vi "DXYN.vi"(11 "Variables and Memory in":T1 {"GFX" format="%02x"}) -> (3 "Variables and Memory out":T1 {"GFX" format="%02x"})   [LabVIEW 2021]
uses:
  Controls/ClusterF.ctl
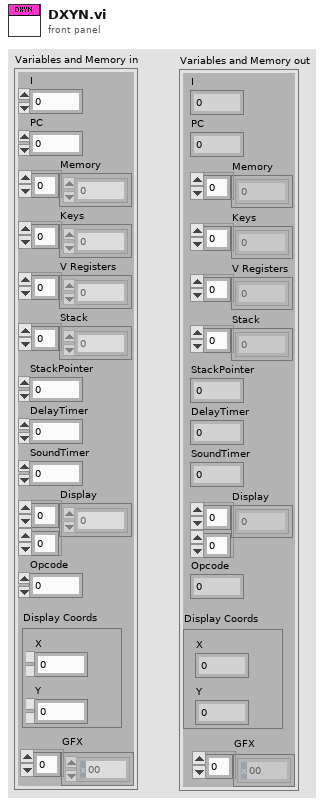
[diagram p1: front panel]
types:
  T1 = typedef "ClusterF.ctl" = cluster{"I":u16, "PC":u16, "Memory":u8[], "Keys":u8[], "V Registers":u8[], "Stack":u16[], "StackPointer":u16, "DelayTimer":u8, "SoundTimer":u8, "Display":u8[][], "Opcode":u16, "Display Coords":cluster{"X":u8, "Y":u8}, "GFX":u8[]}
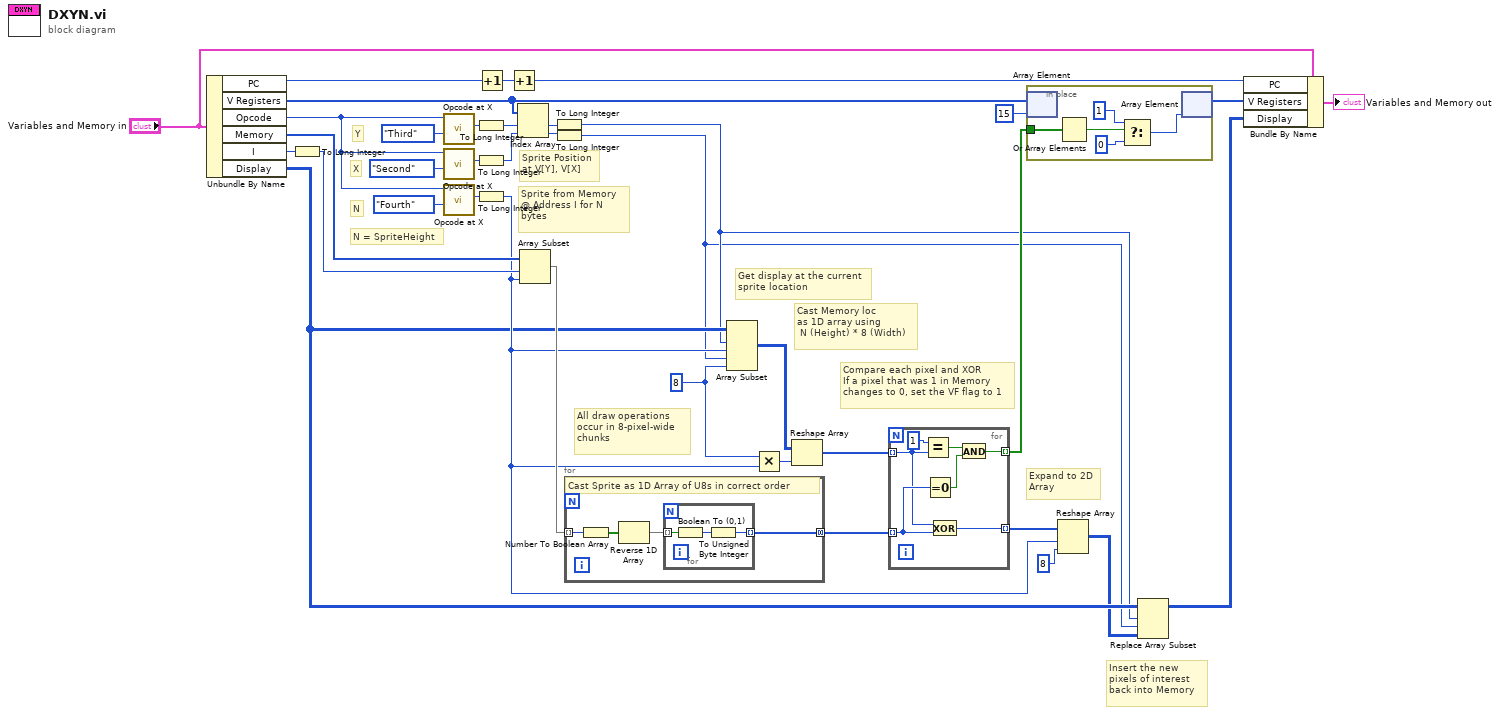
[diagram p0: block diagram]
diagram:
  w13 = 8 ("length")
  # "Insert the new\npixels of interest\nback into Memory"
  # "Expand to 2D\nArray"
  # "Compare each pixel and XOR\nIf a pixel that was 1 in Memory\nchanges to 0, set the VF flag to 1"
  # "Cast Memory loc \nas 1D array using\n N (Height) * 8 (Width)"
  # "Get display at the current\nsprite location"
  # "All draw operations\noccur in 8-pixel-wide\nchunks"
  # "Sprite Position\nat V[Y], V[X]"
  # "Sprite from Memory\n@ Address I for N\nbytes"
  # "N = SpriteHeight"
  # "N"
  # "X"
  # "Y"
  n1 = Unbundle By Name("Variables and Memory in") -> ("PC"=w24:u16, "V Registers"=w29:u8[], "Opcode"=w32:u16, "Memory"=w21:u8[], "I"=w20:u16, "Display"=w5:u8[][])
  n2 = To Long Integer(number=w20) -> (32bit integer=w19:i32)
  n3 = call "Opcode at X.vi"("X Position"=enum16{"First", "Second", "Third", "Fourth"}."Third", "Opcode"=w32) -> ("Opcode at X Position (U8)"=w28:u8)  [unwired: 9 in]
  n4 = call "Opcode at X.vi"("X Position"=enum16{"First", "Second", "Third", "Fourth"}."Second", "Opcode"=w32) -> ("Opcode at X Position (U8)"=w26:u8)  [unwired: 9 in]
  n5 = call "Opcode at X.vi"("X Position"=enum16{"First", "Second", "Third", "Fourth"}."Fourth", "Opcode"=w32) -> ("Opcode at X Position (U8)"=w18:u8)  [unwired: 9 in]
  n6 = To Long Integer(number=w28) -> (32bit integer=w27:i32)
  n7 = To Long Integer(number=w26) -> (32bit integer=w25:i32)
  n8 = To Long Integer(number=w18) -> (32bit integer=w7:i32)
  n9 = Increment(x=w24) -> (x+1=w22:u16)
  n10 = Increment(x=w22) -> (x+1=w23:u16)
  n11 = Index Array(array=w29, index #1=w27, index #2=w25) -> (element #1=w17:u8, element #2=w16:u8)
  n12 = Array Subset(array=w21, index=w19, length=w7) -> (w15:u8[])
  n13 = To Long Integer(number=w17) -> (32bit integer=w4:i32)
  n14 = To Long Integer(number=w16) -> (32bit integer=w3:i32)
  n15 = for {
    tunnel: w15 -> [w41] mode=indexing
    tunnel: [w38] -> w10 mode=concatenating
    # "Cast Sprite as 1D Array of U8s in correct order"
    n16 = Number To Boolean Array(number=w41) -> (Boolean array=w40:bool[])
    n17 = Reverse 1D Array(array=w40) -> (reversed array=w39:bool[])
    n18 = for {
      tunnel: w39 -> [w44] mode=indexing
      tunnel: [w42] -> w38 mode=indexing
      n19 = Boolean To (0,1)(Boolean=w44) -> (0, 1=w43:i16)
      n20 = To Unsigned Byte Integer(number=w43) -> (unsigned 8bit integer=w42:u8)
    }
  }
  n21 = Array Subset(array=w5, index (row)=w4, length (row)=w7, index (col)=w3, length (col)=w13) -> (w14:u8[][])
  n22 = Multiply(x=w13, y=w7) -> (x*y=w12:i32)
  n23 = Reshape Array(w14, w12) -> (w11:u8[])
  n24 = for {
    tunnel: w11 -> [w49] mode=indexing
    tunnel: w10 -> [w50] mode=indexing
    tunnel: [w46] -> w9 mode=indexing
    tunnel: [w45] -> w8 mode=indexing
    n25 = Equal?(x=u8 1, y=w49) -> (x = y?=w48:bool)
    n26 = Equal To 0?(x=w50) -> (x = 0?=w47:bool)
    n27 = Exclusive Or(1:w50, 2:w49) -> (0:w45:u8)
    n28 = And(x=w48, y=w47) -> (x .and. y?=w46:bool)
  }
  n29 = in-place {
    in-place-border: w9 -> [w52]
    n30 = in-place-array #1(w29, 15) -> ()  [unwired: 1 out]
    n31 = Or Array Elements(Boolean array=w52) -> (logical OR=w53:bool)
    n32 = Select(t=u8 1, s=w53, f=u8 0 ("element")) -> (s? t:f=w54:u8)
    n33 = in-place-array #1(w54) -> (w30:u8[])  [unwired: 1 out]
  }
  n34 = Reshape Array(w8, w7, 8 ("dimension size")) -> (w2:u8[][])
  n35 = Replace Array Subset(array=w5, new element=w2, index (row)=w4, index (col)=w3) -> (w1:u8[][])
  n36 = Bundle By Name(cluster="Variables and Memory in", "PC"=w23, "V Registers"=w30, "Display"=w1) -> (→"Variables and Memory out":T1)
